vi "Compare Parameters With Refresh Dialog.vi"(8 "error in":errorcluster, 9 "refresh button":bool, 10 "selected parameters file":path caption="path to parameters xml", 11 "configuration files page data in":T1 {"custom device ref" format="%.0x"}) -> (0 "error out":errorcluster, 3 "configuration files page data out":T1 {"custom device ref" format="%.0x"})   [LabVIEW 2020, in "AIM ARINC 429 System Explorer.lvlib" / "Implementation.lvlib"]
uses:
  Implementation.lvlib
  Import/ARINC 429 Import.lvlib
  Scripting/AIM/AIM ARINC 429 Scripting.lvlib
  Types/Browse Button.ctl
  Types/Path Control.ctl
  <vilib>/NI VeriStand/Custom Device API/Custom Device Item Ref.ctl
  <vilib>/NI VeriStand/Custom Device API/Custom Device API.lvlib
  Types/Configuration Files Page Data.ctl
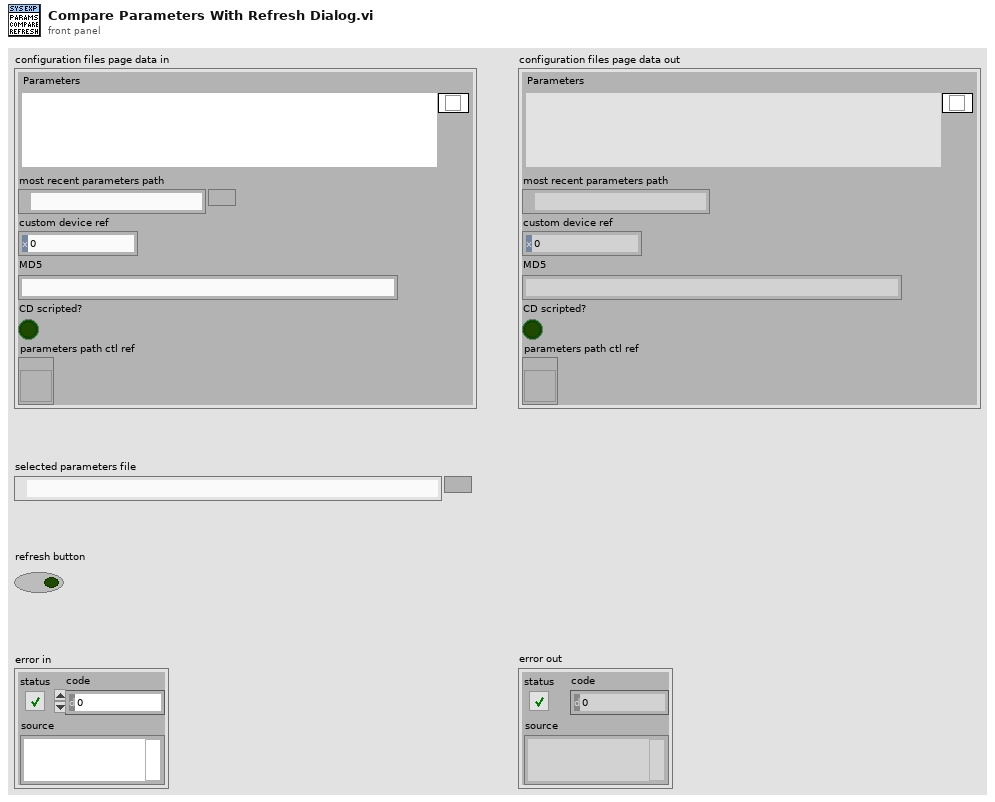
[diagram p1: front panel]
types:
  T1 = typedef "AIM ARINC 429 System Explorer.lvlib/Implementation.lvlib/Configuration Files Page Data.ctl" = cluster{"Parameters":T2, "most recent parameters path":path, "custom device ref":T4, "MD5":string, "CD scripted?":bool, "parameters path ctl ref":refnum<vi>}
  T2 = typedef "AIM ARINC 429 System Explorer.lvlib/Implementation.lvlib/Path Control.ctl" = cluster{"file path":path, "Browse":T3}
  T3 = typedef "AIM ARINC 429 System Explorer.lvlib/Implementation.lvlib/Browse Button.ctl" = bool
  T4 = typedef "Custom Device API.lvlib/Custom Device Item Ref.ctl" = u64
  T5 = typedef "VS Channels Definition for All Labels on Hardware Channel.ctl" = cluster{"hardware channel":i32, "direction":T6, "labels":T7[]}
  T6 = typedef "Direction.ctl" = enum16{"Rx", "Tx"}
  T7 = typedef "VS Channels Definition for Label.ctl" = cluster{"label (Dec)":u32, "parameters":T8[], "SDI value":u8, "SDI enabled":bool, "transfer type":T11, "create timestamp":bool}
  T8 = typedef "VS Channel Definition for Parameter.ctl" = cluster{"name":string, "default value":dbl, "unit":string, "Parameter":T9}
  T9 = typedef "Parameter Definition.ctl" = cluster{"start index":i32, "size":i32, "encoding":T10, "signed":bool, "scale multiplier":dbl, "scale offset":dbl}
  T10 = typedef "Encoding and Decoding.lvlib/Encoding.ctl" = enum16{"BNR", "BCD", "Discrete"}
  T11 = typedef "Transfer Type.ctl" = enum16{"Scheduled", "Acyclic", "Block", "Strobe"}
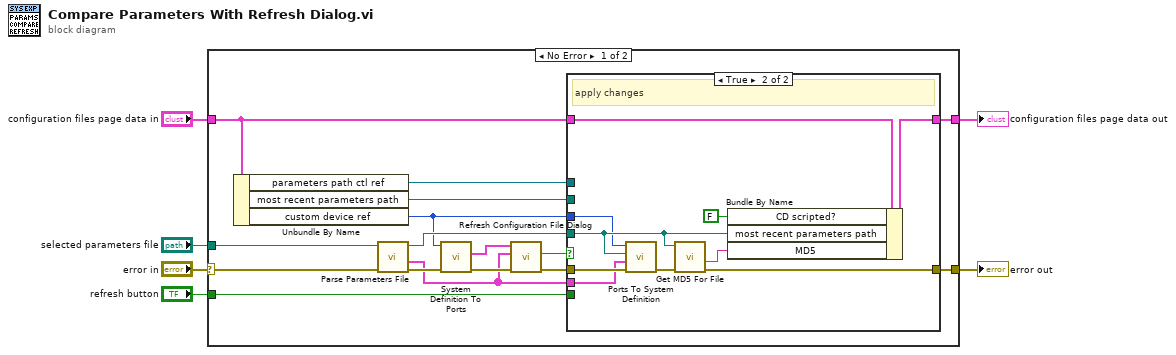
[diagram p0: block diagram]
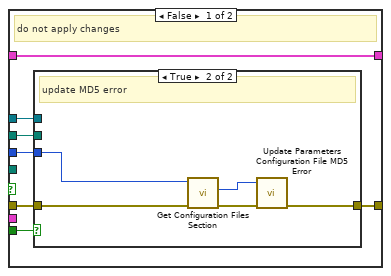
[diagram p2: hidden frame]
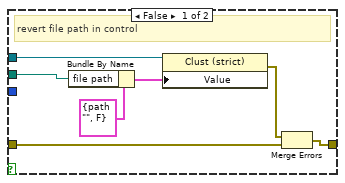
[diagram p3: hidden frame]
diagram:
  n1 = case shown="No Error" "error in" {
    selector: "error in" -> [w22 w53]
    tunnel: [w21 w53] -> w5
    tunnel: "configuration files page data in" -> [w19 w52]
    tunnel: [w18 w52] -> w3
    tunnel: "selected parameters file" -> [w20 _]
    tunnel: "refresh button" -> [w17 _]
    frame No Error {
      n2 = Unbundle By Name(w19) -> ("parameters path ctl ref"=w7:refnum<vi>, "most recent parameters path"=w8:path, "custom device ref"=w9:T4)
      n3 = call "Parse Parameters File.vi"("error in"=w22, "path to XML document"=w20) -> ("error out"=w16:errorcluster, "ports"=w10:T5[], "path to XML document out"=w11:path)  [unwired: 7 in]
      n4 = call "System Definition To Ports.vi"("error in"=w16, "custom device ref"=w9) -> ("error out"=w15:errorcluster, "ports"=w14:T5[])  [unwired: 7 in, 1 out]
      n5 = call "Refresh Configuration File Dialog.vi"("error in"=w15, "new ports"=w10, "current ports"=w14) -> ("error out"=w12:errorcluster, "apply changes"=w13:bool)  [unwired: 7 in]
      n6 = case shown="True" w13 {
        tunnel: w12 -> [w28 w51]
        tunnel: w11 -> [_ w45]
        tunnel: w10 -> [_ w50]
        tunnel: [w29 w46] -> w21
        tunnel: w19 -> [w27 w48]
        tunnel: [w27 w49] -> w18
        tunnel: w17 -> [w26 _]
        tunnel: w9 -> [w25 w43]
        tunnel: w8 -> [w24 _]
        tunnel: w7 -> [w23 _]
        frame False {
          # "do not apply changes"
          n7 = case shown="True" w26 {
            tunnel: [w34 w39] -> w29
            tunnel: w28 -> [w32 w38]
            tunnel: w25 -> [_ w37]
            tunnel: w24 -> [w31 _]
            tunnel: w23 -> [w30 _]
            frame False {
              # "revert file path in control"
              n8 = Bundle By Name(cluster=T2 {"file path"=path "", "Browse"=FALSE} ("Value"), "file path"=w31) -> (w35:T2)
              n9 = property class="Clust (strict)"(reference=w30, "Value"=w35) -> (error out=w33:errorcluster)  [unwired: 1 in, 1 out]
              n10 = Merge Errors(w33, w32) -> (w34:errorcluster)
            }
            frame True {
              # "update MD5 error"
              n11 = call "Get Configuration Files Section.vi"("error in"=w38, "Custom device Ref"=w37) -> ("error out"=w40:errorcluster, "Configuration files Ref"=w41:T4)  [unwired: 7 in, 1 out]
              n12 = call "Update Parameters Configuration File MD5 Error.vi"("error in"=w40, "configuration files ref"=w41) -> ("error out"=w39:errorcluster)  [unwired: 8 in, 1 out]
            }
          }
        }
        frame True {
          # "apply changes"
          n13 = call "Ports To System Definition.vi"("error in"=w51, "ports"=w50, "parameter configuration file path"=w45, "custom device ref"=w43) -> ("error out"=w47:errorcluster)  [unwired: 6 in, 1 out]
          n14 = call "Get MD5 For File.vi"("error in"=w47, "path"=w45) -> ("error out"=w46:errorcluster, "MD5"=w44:string)  [unwired: 8 in]
          n15 = Bundle By Name(cluster=w48, "CD scripted?"=FALSE, "most recent parameters path"=w45, "MD5"=w44) -> (w49:T1)
        }
      }
    }
    frame Error {
    }
  }
  "error out" <- w5
  "configuration files page data out" <- w3
